vi "Open PID Ref.vi"() -> (0 "error out":errorcluster, 3 "VI out":refnum<vi>)   [LabVIEW 2024]
uses:
  <vilib>/addons/control/pid/pid.llb/PID (DBL).vi
  <vilib>/addons/control/pid/NI_PID_pid.lvlib
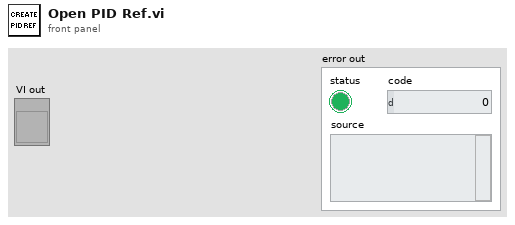
[diagram p1: front panel]
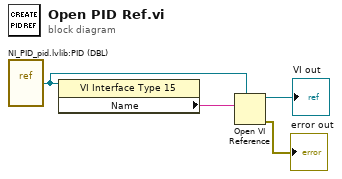
[diagram p0: block diagram]
diagram:
  n1 = vi-ref "NI_PID_pid.lvlib:PID (DBL).vi"() -> (w3:refnum<vi>)
  n2 = property class="VI Interface Type 15"(reference=w3) -> ("Name"=w2:string)  [unwired: 1 in, 2 out]
  n3 = Open VI Reference(type specifier VI Refnum (for type only)=w3, vi path=w2) -> (vi reference=→"VI out":refnum<vi>, error out=→"error out":errorcluster)  [unwired: 4 in]
